vi "initialise.vi"(3 "Reset Device (Reset Device)":i16, 4 "ID Query (Do Query)":i16, 5 "resource name":string="USB0::0x1313::0x8078::P0005368::INSTR") -> (0 "error out":errorcluster {"code" format="%.0x"}, 2 "instrument handle out":refnum<visa-resource-name>)   [LabVIEW 2015]
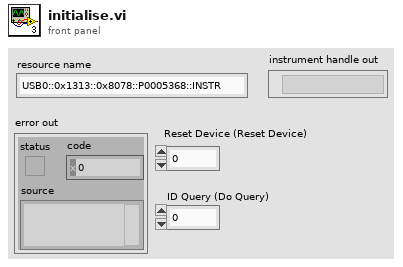
[diagram p1: front panel]
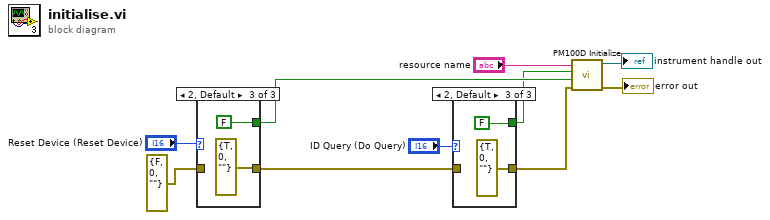
[diagram p0: block diagram]
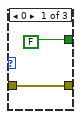
[diagram p2: hidden frame]
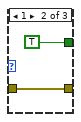
[diagram p3: hidden frame]
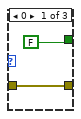
[diagram p4: hidden frame]
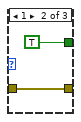
[diagram p5: hidden frame]
diagram:
  n1 = case shown="2, Default" "Reset Device (Reset Device)" {
    tunnel: [FALSE TRUE FALSE] -> w6
    tunnel: [w11 w13 errorcluster {"status"=TRUE, "code"=0, "source"=""} ("error in (no error)")] -> w4
    tunnel: errorcluster {"status"=FALSE, "code"=0, "source"=""} ("error in (no error)") -> [w11 w13 _]
    frame 0 {
    }
    frame 1 {
    }
    frame 2, Default {
    }
  }
  n2 = case shown="2, Default" "ID Query (Do Query)" {
    tunnel: [FALSE TRUE FALSE] -> w3
    tunnel: [w17 w19 errorcluster {"status"=TRUE, "code"=0, "source"=""} ("error in (no error)")] -> w2
    tunnel: w4 -> [w17 w19 _]
    frame 0 {
    }
    frame 1 {
    }
    frame 2, Default {
    }
  }
  n3 = call "PM100D Initialize.vi"("error in (no error)"=w2, "Reset Device (Reset Device)"=w6, "ID Query (Do Query)"=w3, "resource name"="resource name") -> ("error out"=→"error out":errorcluster, "instrument handle out"=→"instrument handle out":refnum<visa-resource-name>)  [unwired: 6 in]
